vi "Video Wait.vi"(8 "error in (no error)":errorcluster, 11 "Ctl Refs in":T1) -> (0 "error out":errorcluster, 3 "Ctl Refs out":T1)   [LabVIEW 2013]
uses:
  Controls/Refs.ctl
  Controls/Button Refs.ctl
  Controls/Tab Ctl Refs.ctl
  types/TabStateType.ctl
  Controls/Indicator Refs.ctl
  Controls/Slider Refs.ctl
  Controls/Control Refs.ctl
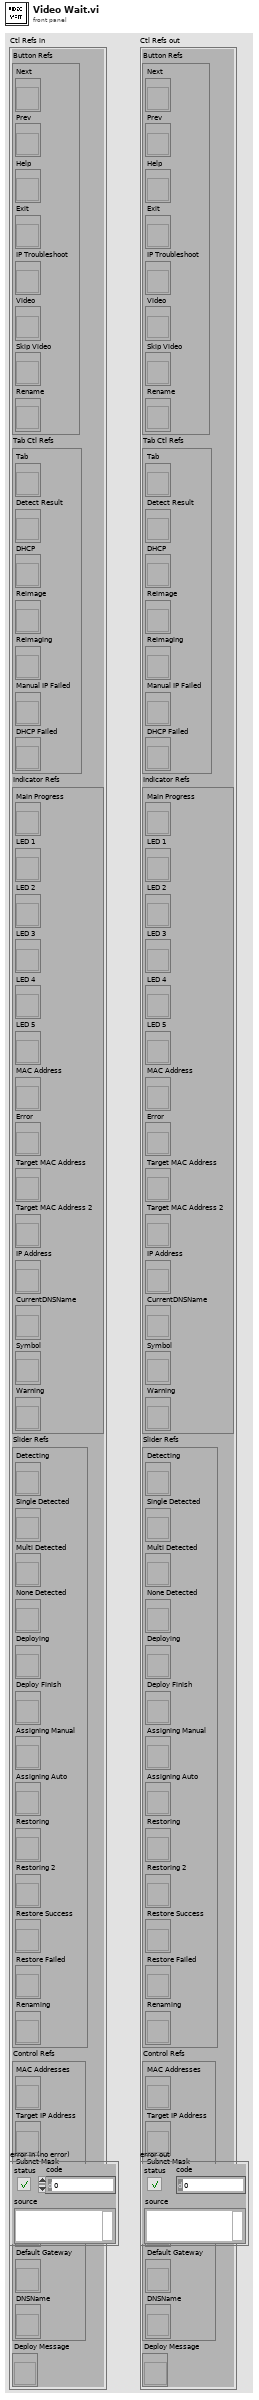
[diagram p1: front panel]
types:
  T1 = typedef "Refs.ctl" = cluster{"Button Refs":T2, "Tab Ctl Refs":T3, "Indicator Refs":T4, "Slider Refs":T5, "Control Refs":T6, "Deploy Message":refnum<vi>}
  T2 = typedef "Button Refs.ctl" = cluster{"Next":refnum<vi>, "Prev":refnum<vi>, "Help":refnum<vi>, "Exit":refnum<vi>, "IP Troubleshoot":refnum<vi>, "Video":refnum<vi>, "Skip Video":refnum<vi>, "Rename":refnum<vi>}
  T3 = typedef "Tab Ctl Refs.ctl" = cluster{"Tab":refnum<vi>, "Detect Result":refnum<vi>, "DHCP":refnum<vi>, "Reimage":refnum<vi>, "Reimaging":refnum<vi>, "Manual IP Failed":refnum<vi>, "DHCP Failed":refnum<vi>}
  T4 = typedef "Indicator Refs.ctl" = cluster{"Main Progress":refnum<vi>, "LED 1":refnum<vi>, "LED 2":refnum<vi>, "LED 3":refnum<vi>, "LED 4":refnum<vi>, "LED 5":refnum<vi>, "MAC Address":refnum<vi>, "Error":refnum<vi>, "Target MAC Address":refnum<vi>, "Target MAC Address 2":refnum<vi>, "IP Address":refnum<vi>, "CurrentDNSName":refnum<vi>, "Symbol":refnum<vi>, "Warning":refnum<vi>}
  T5 = typedef "Slider Refs.ctl" = cluster{"Detecting":refnum<vi>, "Single Detected":refnum<vi>, "Multi Detected":refnum<vi>, "None Detected":refnum<vi>, "Deploying":refnum<vi>, "Deploy Finish":refnum<vi>, "Assigning Manual":refnum<vi>, "Assigning Auto":refnum<vi>, "Restoring":refnum<vi>, "Restoring 2":refnum<vi>, "Restore Success":refnum<vi>, "Restore Failed":refnum<vi>, "Renaming":refnum<vi>}
  T6 = typedef "Control Refs.ctl" = cluster{"MAC Addresses":refnum<vi>, "Target IP Address":refnum<vi>, "Subnet Mask":refnum<vi>, "DNS IP":refnum<vi>, "Default Gateway":refnum<vi>, "DNSName":refnum<vi>}
  T7 = enum32{"Welcome", "Instructions", "Detect", "Run Detection", "Detect Result", "Deploy", "Run Deployment", "Connect Verify", "Success", "DHCP", "Troubleshoot", "System Restore", "Error", "Video"}
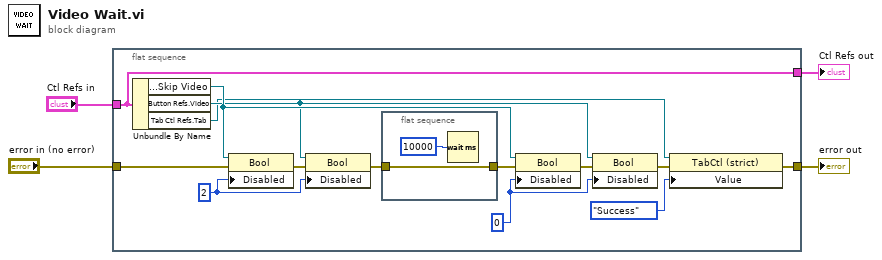
[diagram p0: block diagram]
diagram:
  n1 = flat-sequence {
    tunnel: [w18] -> w1
    tunnel: "error in (no error)" -> [w15]
    tunnel: "Ctl Refs in" -> [w5]
    tunnel: [w5] -> w4
    frame #0 {
      w9 = u8 0 ("Disabled")
      w13 = u8 2 ("Disabled")
      n2 = Unbundle By Name(w5) -> ("Button Refs.Skip Video"=w8:refnum<vi>, "Button Refs.Video"=w7:refnum<vi>, "Tab Ctl Refs.Tab"=w6:refnum<vi>)
      n3 = property on="Property Node" class="Bool"(reference=w8, error in=w15, "Disabled"=w13) -> (error out=w16:errorcluster)  [unwired: 1 out]
      n4 = property on="Property Node" class="Bool"(reference=w7, error in=w16, "Disabled"=w13) -> (error out=w14:errorcluster)  [unwired: 1 out]
      n5 = flat-sequence {
        tunnel: w14 -> [w20]
        tunnel: [w20] -> w12
        frame #0 {
          n6 = Wait (ms)(milliseconds to wait=u32 10000) -> ()  [unwired: 1 out]
        }
      }
      n7 = property on="Property Node" class="Bool"(reference=w8, error in=w12, "Disabled"=w9) -> (error out=w11:errorcluster)  [unwired: 1 out]
      n8 = property on="Property Node" class="Bool"(reference=w7, error in=w11, "Disabled"=w9) -> (error out=w10:errorcluster)  [unwired: 1 out]
      n9 = property on="Property Node" class="TabCtl (strict)"(reference=w6, error in=w10, "Value"=T7."Success" ("Tab Control")) -> (error out=w18:errorcluster)  [unwired: 1 out]
    }
  }
  "Ctl Refs out" <- w4
  "error out" <- w1
